vi "Read Modules URLs.vi"(8 "error in":errorcluster, 11 "Engine Parent in":refnum<class "Engine Parent Editor Node.lvclass">) -> (0 "error out":errorcluster, 2 "components URLs":string[](array[string]), 3 "Engine Parent out":refnum<class "Engine Parent Editor Node.lvclass">)   [LabVIEW 2013, in "PL Framework Configuration Tool.lvlib" / "Engine Parent Editor Node.lvclass"]
uses:
  Engine Parent Editor Node.lvclass
  <vilib>/NI/CEF/CEF_TreeControl/Node/NISE_CEF_Node.lvclass/NISE_CEF_Node.ctl
  Module editor node/module editor node.lvclass
  <vilib>/NI/Tag Bus/tag/tag descriptor.lvclass/tag descriptor.ctl
  <vilib>/NI/CEF/CEF_TreeControl/Node/NISE_CEF_Node.lvclass
  <vilib>/NI/Tag Bus Module Framework/module configuration/TBM module configuration.lvclass
  <vilib>/NI/Tag Bus/tag/tag descriptor.lvclass
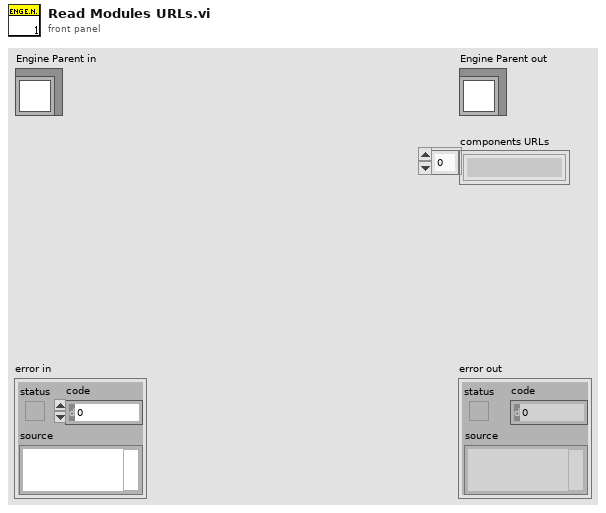
[diagram p1: front panel]
types:
  T1 = typedef "NISE_CEF_Node.lvclass/NodeRef.ctl" = refnum<data-value>
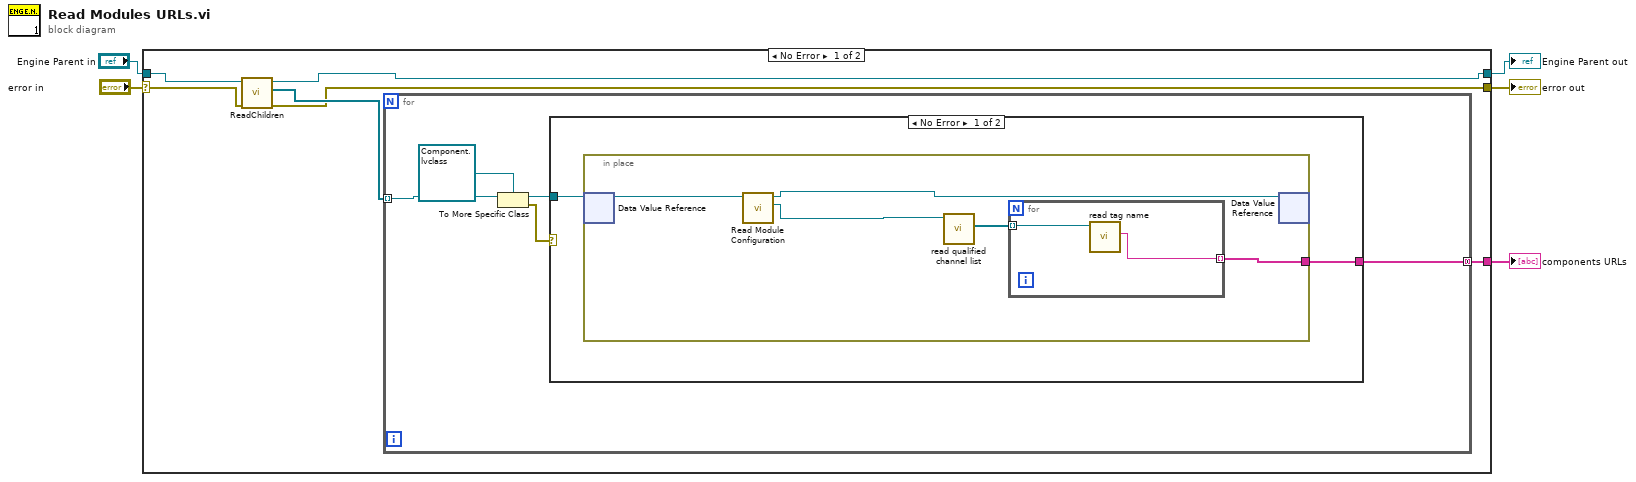
[diagram p0: block diagram]
diagram:
  n1 = case shown="No Error" "error in" {
    selector: "error in" -> [w6 w26]
    tunnel: [w7 w26] -> w3
    tunnel: [w8 w27] -> w4
    tunnel: "Engine Parent in" -> [w10 w27]
    tunnel: [w11 _] -> w5
    frame No Error {
      n2 = call <vilib>:"ReadChildren.vi"("error in"=w6, "node in"=w10) -> ("error out"=w7:errorcluster, "output array"=w9:T1[], "node out"=w8:refnum<class "Engine Parent Editor Node.lvclass">)  [unwired: 7 in]
      n3 = for {
        tunnel: [w16] -> w11 mode=concatenating
        tunnel: w9 -> [w13] mode=indexing
        n4 = To More Specific Class(target class=refnum<data-value> refnum ("data value reference"), reference=w13) -> (specific class reference=w15:refnum<data-value>, error out=w14:errorcluster)  [unwired: 1 in]
        n5 = case shown="No Error" w14 {
          tunnel: [w18 _] -> w16
          tunnel: w15 -> [w17 _]
          frame No Error {
            n6 = in-place {
              in-place-border: [w23] -> w18
              n7 = in-place-dvr #1(w17) -> (w22:refnum<class "module editor node.lvclass">)  [unwired: 1 out]
              n8 = call "Read Module Configuration.vi"("Module Editor Node in"=w22) -> ("module configuration"=w19:refnum<class "TBM module configuration.lvclass">, "Module Editor Node out"=w21:refnum<class "module editor node.lvclass">)  [unwired: 8 in, 1 out]
              n9 = call <vilib>:"read qualified channel list.vi"("module configuration in"=w19) -> ("qualified channels"=w20:refnum<class "TBM channel.lvclass">[])  [unwired: 9 in, 1 out]
              n10 = for {
                tunnel: w20 -> [w25] mode=indexing
                tunnel: [w24] -> w23 mode=indexing
                n11 = call <vilib>:"read tag name.vi"("system tag in"=w25) -> ("name"=w24:string)  [unwired: 8 in, 2 out]
              }
              n12 = in-place-dvr #1(w21) -> ()  [unwired: 2 out]
            }
          }
          frame Error {
          }
        }
      }
    }
    frame Error {
    }
  }
  "error out" <- w3
  "Engine Parent out" <- w4
  "components URLs" <- w5
